vi "Polynomials Composition (DBL).vi"(8 "threshold type":T1 items=["Absolute Value", "Relative Value"], 9 "threshold":dbl, 10 "Q(x)":dbl[](array[numeric]), 11 "P(x)":dbl[](array[numeric])) -> (0 "error":i32, 3 "P(Q(x))":dbl[](array[numeric]))   [LabVIEW 2020, in "NI_AALPro.lvlib"]
doc: "Computes the composition of polynomials <B>P(x)</B> and <B>Q(x)</B>. The data types you wire to the <B>P(x)</B> and <B>Q(x)</B> inputs determine the polymorphic instance to use."
uses:
  <vilib>/Analysis/NI_AALPro.lvlib
  <vilib>/Analysis/polynomials.llb/Remove Zero Threshold Type.ctl
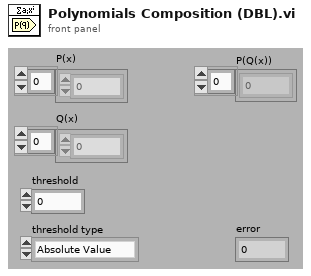
[diagram p1: front panel]
types:
  T1 = typedef "NI_AALPro.lvlib/Remove Zero Threshold Type.ctl" = u16
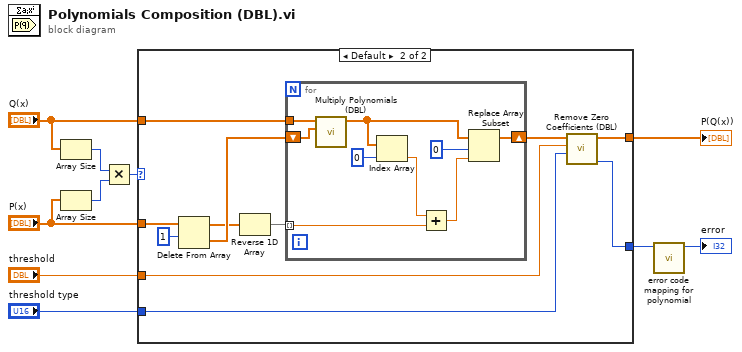
[diagram p0: block diagram]
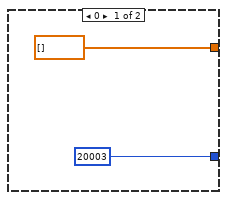
[diagram p2: hidden frame]
diagram:
  n1 = Array Size(array="Q(x)") -> (size(s)=w7:i32)
  n2 = Array Size(array="P(x)") -> (size(s)=w6:i32)
  n3 = Multiply(x=w7, y=w6) -> (x*y=w5:i32)
  n4 = case shown="Default" w5 {
    tunnel: "P(x)" -> [_ w23]
    tunnel: "Q(x)" -> [_ w20]
    tunnel: [dbl[] [] ("BDL") w19] -> w10
    tunnel: [20003 ("empty array") w15] -> w4
    tunnel: "threshold" -> [_ w14]
    tunnel: "threshold type" -> [_ w13]
    frame 0 {
    }
    frame Default {
      n5 = Delete From Array(array=w23, length=1) -> (deleted portion=w22:dbl[], array with subset deleted=w16:dbl[])  [unwired: 1 in]
      n6 = Reverse 1D Array(array=w16) -> (reversed array=w17:dbl[])
      n7 = for {
        tunnel: w17 -> [w29] mode=indexing
        tunnel: w20 -> [w32]
        shift-right: [w26] -> w18
        shift-left: w22 -> [w31]
        n8 = call <vilib>:"Multiply Polynomials (DBL).vi"("Q(x)"=w31, "P(x)"=w32) -> ("P(x)*Q(x)"=w27:dbl[])  [unwired: 8 in, 1 out]
        n9 = Index Array(array=w27, index=0) -> (element=w30:dbl)
        n10 = Add(x=w30, y=w29) -> (x+y=w28:dbl)
        n11 = Replace Array Subset(array=w27, new element=w28, index=0) -> (w26:dbl[])
      }
      n12 = call <vilib>:"Remove Zero Coefficients (DBL).vi"("threshold type"=w13, "threshold"=w14, "P(x) In"=w18) -> ("error"=w15:i32, "P(x) Out"=w19:dbl[])  [unwired: 6 in, 1 out]
    }
  }
  "P(Q(x))" <- w10
  n13 = call <vilib>:"error code mapping for polynomial.vi"("error in"=w4) -> ("error out"=→"error":i32)  [unwired: 10 in]
